vi "MCL Filter Mixed Mode Data.vi"(10 "Data":dbl[][](array[numeric])) -> (2 "Mixed Mode Data":T1[](array[typedef]))   [LabVIEW 2013]
uses:
  MixedMode/Mixed Mode Cartesian Data.ctl
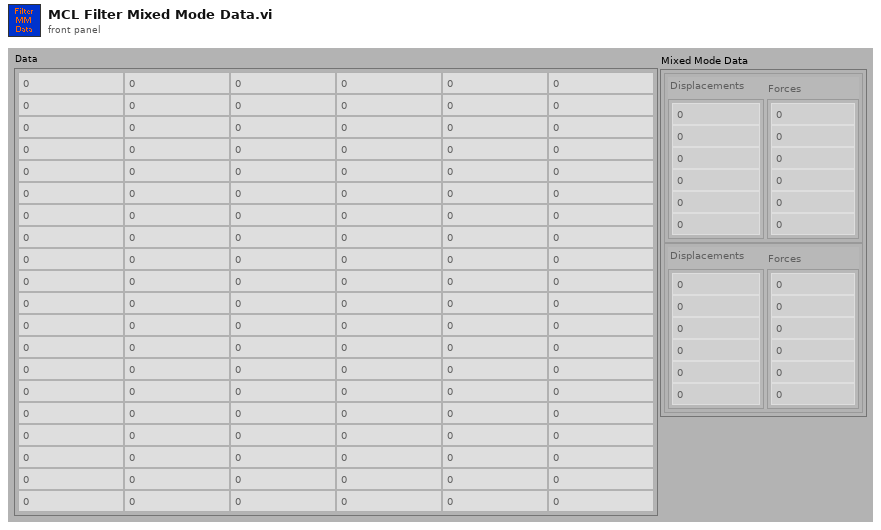
[diagram p1: front panel]
types:
  T1 = typedef "Mixed Mode Cartesian Data.ctl" = cluster{"Displacements":dbl[], "Forces":dbl[]}
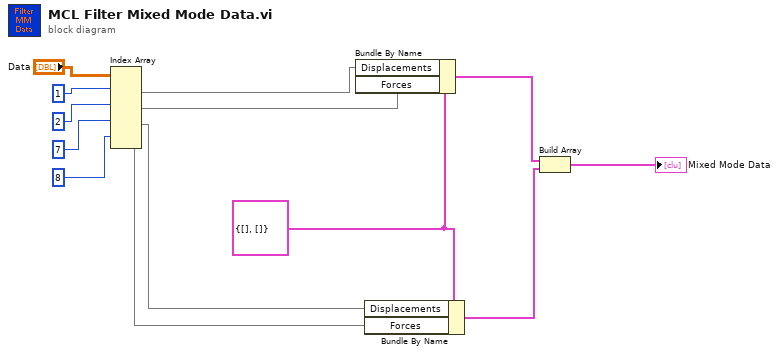
[diagram p0: block diagram]
diagram:
  w13 = T1 {"Displacements"=[], "Forces"=[]} ("LBCB 1 Measurements")
  n1 = Index Array(array="Data", index (row) #1=1 ("index (row)"), index (row) #2=2 ("index (row)"), index (row) #3=7 ("index (row)"), index (row) #4=8 ("index (row)")) -> (element #1=w7:dbl[], element #2=w2:dbl[], element #3=w1:dbl[], element #4=w6:dbl[])  [unwired: 4 in]
  n2 = Bundle By Name(cluster=w13, "Displacements"=w7, "Forces"=w2) -> (w5:T1)
  n3 = Bundle By Name(cluster=w13, "Displacements"=w1, "Forces"=w6) -> (w4:T1)
  n4 = Build Array(w5, w4) -> (→"Mixed Mode Data":T1[])
